vi "Add undelivered instance.vi"(5 "Year":i32, 7 "Month":i32, 8 "Error In":errorcluster, 10 "Dates in":timestamp[](array[timestamp]), 11 "INI Ref in":T2) -> (0 "Error Out":errorcluster, 1 "User":string, 2 "Original instance":string, 3 "INI Ref out":T2, 4 "Cancelled?":bool, 6 "Paper instance":T1)   [LabVIEW 2015]
uses:
  <vilib>/Utility/config.llb/Config Data RefNum.ctl
  Home/Undelivered instance.ctl
  Undelivered state.ctl
  <vilib>/Utility/config.llb/NI_LVConfig.lvlib
panel:
  in  "Cancel":bool
  in  "OK":bool
  in  "Help string":bool
  in  "Instances":string
  in  "Newspaper name":string(combo)
  # "Select the newspaper for which you want to enter an instance of a missed delivery, and then type in the instances of missing deliveries. Click Help to see the ways you can enter instances."
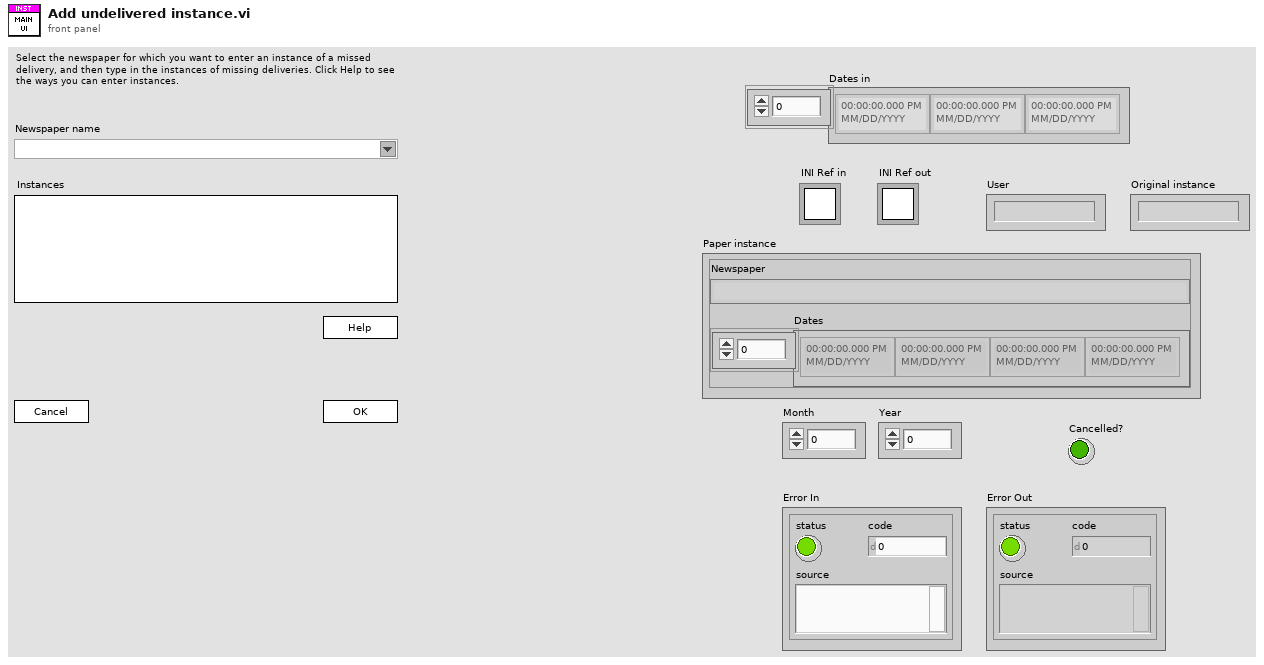
[diagram p1: front panel]
types:
  T1 = typedef "Undelivered instance.ctl" = cluster{"Dates":timestamp[], "Newspaper":string}
  T2 = typedef "NI_LVConfig.lvlib/Config Data RefNum.ctl" = refnum<k1>
  T3 = typedef "Undelivered state.ctl" = enum16{"Init", "Idle", "Check instance string", "Show help", "Exit"}
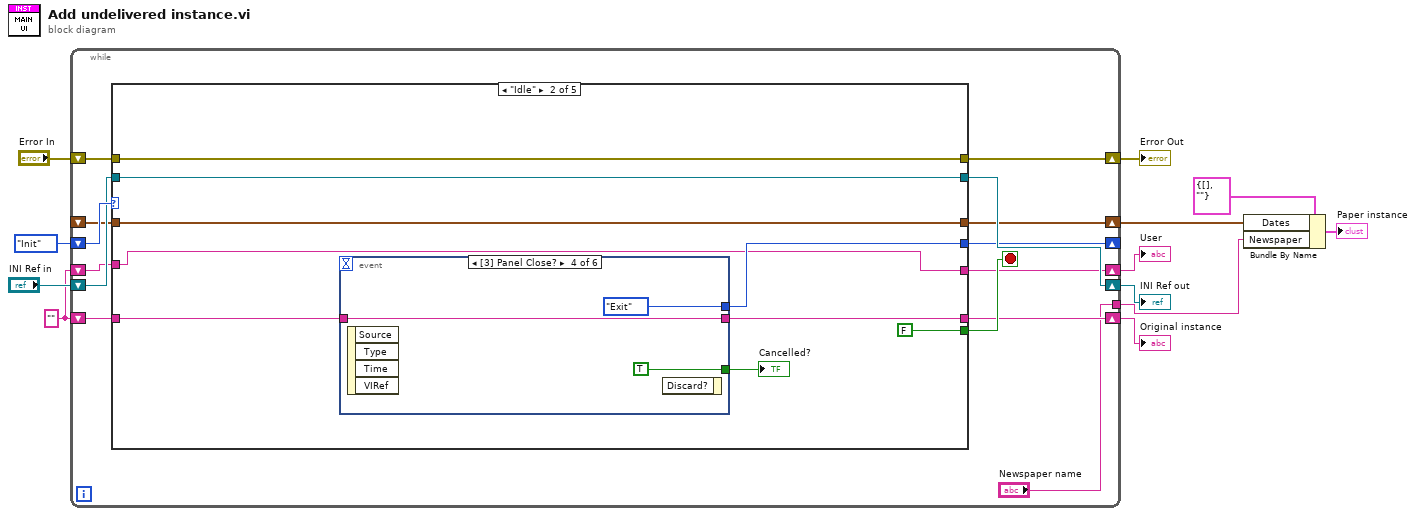
[diagram p0: block diagram]
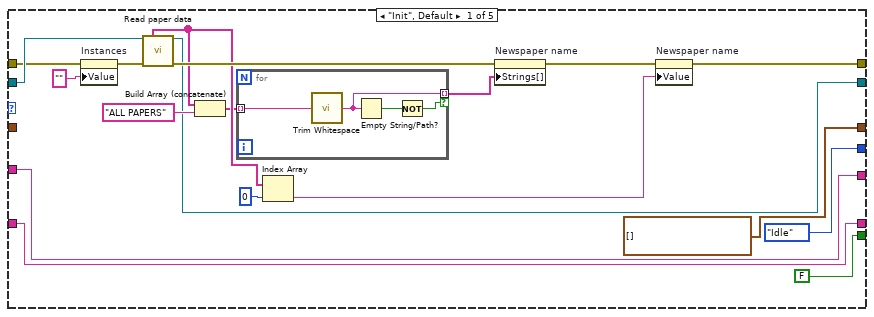
[diagram p2: hidden frame]
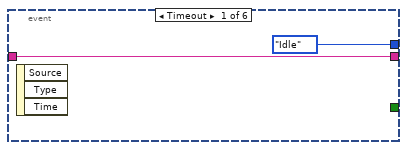
[diagram p3: hidden frame]
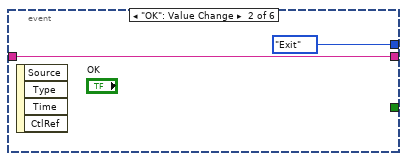
[diagram p4: hidden frame]
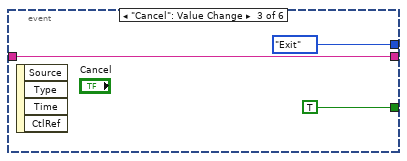
[diagram p5: hidden frame]
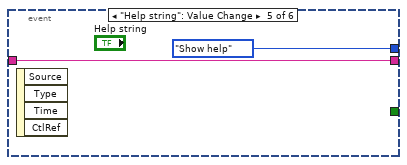
[diagram p6: hidden frame]
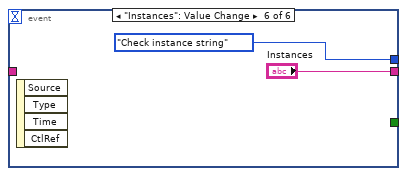
[diagram p7: hidden frame]
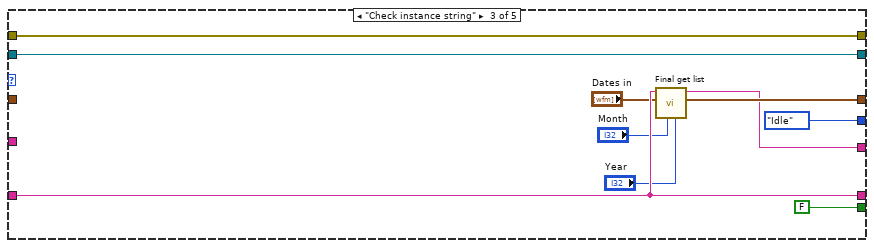
[diagram p8: hidden frame]
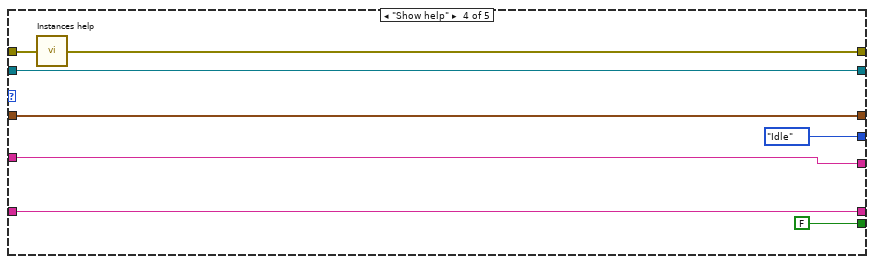
[diagram p9: hidden frame]
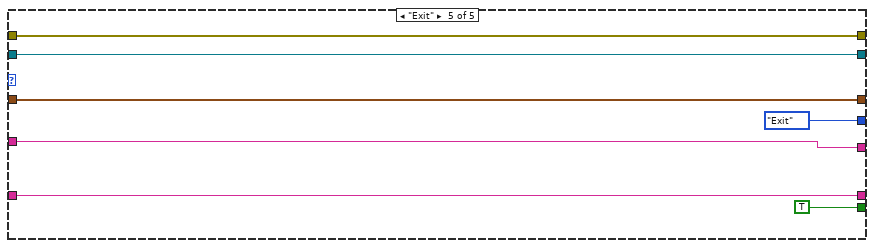
[diagram p10: hidden frame]
diagram:
  w7 = ""
  n1 = while {
    shift-right: [w23] -> w11
    shift-left: "INI Ref in" -> [w25]
    shift-right: [w22] -> w9
    shift-left: "Error In" -> [w24]
    shift-right: [w20] -> _
    shift-left: Undelivered_state."Init" -> [w26]
    shift-right: [w18] -> w1
    shift-left: w7 -> [w19]
    shift-right: [w17] -> w5
    shift-left: _ -> [w14]
    shift-right: [w15] -> w2
    shift-left: w7 -> [w16]
    tunnel: ["Newspaper name"] -> w4
    stop <- w21 stop-if-true
    n2 = case shown="\"Idle\"" w26 {
      tunnel: w25 -> [w45 w50 w76 w85 w96]
      tunnel: w24 -> [w44 w51 w77 w90 w95]
      tunnel: [w37 w50 w76 w85 w96] -> w23
      tunnel: [w36 w51 w77 w88 w95] -> w22
      tunnel: [FALSE FALSE FALSE FALSE TRUE] -> w21
      tunnel: [Undelivered_state."Idle" w58 Undelivered_state."Idle" Undelivered_state."Idle" Undelivered_state."Exit"] -> w20
      tunnel: w19 -> [w31 w54 w82 w86 w91]
      tunnel: [w31 w55 w82 w86 w91] -> w18
      tunnel: [timestamp[] [] ("Dates in") w52 w80 w89 w93] -> w17
      tunnel: w16 -> [w32 w56 _ w87 w92]
      tunnel: [w32 w56 w79 w87 w92] -> w15
      tunnel: w14 -> [_ w52 _ w89 w93]
      frame "Init", Default {
        n3 = property on="Instances" class="Str"(error in=w44, "Value"="" ("Instances")) -> (error out=w28:errorcluster)  [unwired: 1 in, 1 out]
        n4 = call "Read paper data.vi"("Refnum in"=w45, "error in (no error)"=w28) -> ("Names"=w40:string[], "Refnum out"=w37:T2, "error out"=w42:errorcluster)  [unwired: 9 in, 2 out]
        n5 = Build Array (concatenate)(w40, "ALL PAPERS") -> (w30:string[])
        n6 = for {
          tunnel: w30 -> [w49] mode=indexing
          tunnel: [w48] -> w29 mode=indexing if=w46
          n7 = call <vilib>:"Trim Whitespace.vi"("string"=w49) -> ("trimmed string"=w48:string)  [unwired: 1 in]
          n8 = Empty String/Path?(string/path=w48) -> (empty?=w47:bool)
          n9 = Not(x=w47) -> (.not. x?=w46:bool)
        }
        n10 = Index Array(array=w40, index=0) -> (element=w38:string)
        n11 = property on="Newspaper name" class="CmbBox"(error in=w42, "Strings[]"=w29) -> (error out=w41:errorcluster)  [unwired: 1 in, 1 out]
        n12 = property on="Newspaper name" class="CmbBox"(error in=w41, "Value"=w38) -> (error out=w36:errorcluster)  [unwired: 1 in, 1 out]
      }
      frame "Idle" {
        n13 = event shown="[3] Panel Close?" {
          selector: _ -> [_ _ _ _ _ _]
          dyn-events: _ -> [_ _ _ _ _ _]
          timeout: _ -> [_ _ _ _ _ _]
          tunnel: [Undelivered_state."Idle" Undelivered_state."Exit" Undelivered_state."Exit" Undelivered_state."Exit" Undelivered_state."Show help" Undelivered_state."Check instance string"] -> w58
          tunnel: [w59 w62 w63 w66 w69 "Instances"] -> w55
          tunnel: w54 -> [w59 w62 w63 w66 w69 _]
          tunnel: [_ _ TRUE TRUE _ _] -> w53
          event Timeout {
            n14 = event-data() -> ()  [unwired: 1 in, 3 out]
          }
          event "OK": Value Change {
            n15 = event-data() -> ()  [unwired: 1 in, 4 out]
          }
          event "Cancel": Value Change {
            n16 = event-data() -> ()  [unwired: 1 in, 4 out]
          }
          event Panel Close? {
            n17 = event-data() -> ()  [unwired: 1 in, 4 out]
            n18 = event-data() -> ()  [unwired: 2 in, 1 out]
          }
          event "Help string": Value Change {
            n19 = event-data() -> ()  [unwired: 1 in, 4 out]
          }
          event "Instances": Value Change {
            n20 = event-data() -> ()  [unwired: 1 in, 4 out]
          }
        }
        "Cancelled?" <- w53
      }
      frame "Check instance string" {
        n21 = call "Final get list.vi"("Year"="Year", "Month"="Month", "Dates in in"="Dates in", "Instances"=w82) -> ("Dates out"=w80:timestamp[], "User string"=w79:string)  [unwired: 6 in]
      }
      frame "Show help" {
        n22 = call "Instances help.vi"("Error In"=w90) -> ("Error Out"=w88:errorcluster)
      }
      frame "Exit" {
      }
    }
  }
  "Error Out" <- w9
  "INI Ref out" <- w11
  "User" <- w2
  "Original instance" <- w1
  n23 = Bundle By Name(cluster=T1 {"Dates"=[], "Newspaper"=""} ("Paper instance 2"), "Dates"=w5, "Newspaper"=w4) -> (→"Paper instance":T1)
